vi "Get RX Data Width.vi"(8 "error in":errorcluster, 11 "eye scan in":refnum<class "niHighSpeedSerial Eye Scan v1 Host.lvclass">) -> (0 "error out":errorcluster, 2 "rx internal data width":T1=enum."32 Bit", 3 "eye scan out":refnum<class "niHighSpeedSerial Eye Scan v1 Host.lvclass">)   [LabVIEW 2015, in "niHighSpeedSerial Eye Scan v1 Host.lvclass"]
uses:
  <instrlib>/niHighSpeedSerial/Eye Scan/v1/Host/Eye Scan/niHighSpeedSerial Eye Scan v1 Host.lvclass
  <instrlib>/niHighSpeedSerial/Eye Scan/v1/Host/Common/Public/Data Width.ctl
  <instrlib>/niHighSpeedSerial/Eye Scan/v1/Host/Eye Scan/niHighSpeedSerial Eye Scan v1 Host.lvclass/niHighSpeedSerial Eye Scan v1 Host.ctl
  <vilib>/Utility/error.llb/Error Cluster From Error Code.vi
  <vilib>/ErrorRing/Error Ring.xnode
  <instrlib>/niHighSpeedSerial/Eye Scan/v1/Host/Common/niHighSpeedSerial Eye Scan Common v1 Host.lvlib
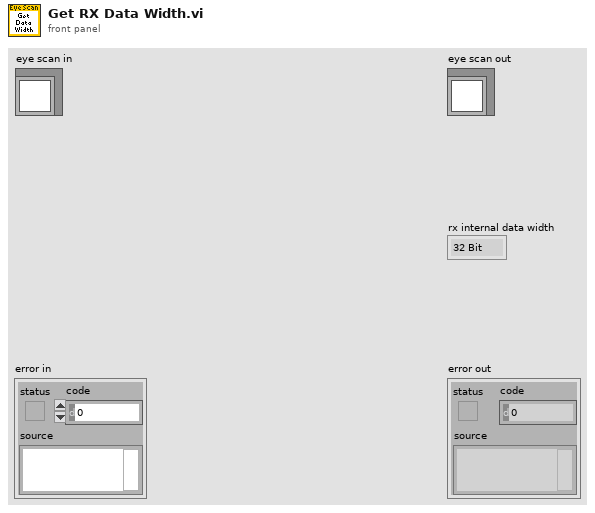
[diagram p1: front panel]
types:
  T1 = typedef "niHighSpeedSerial Eye Scan Common v1 Host.lvlib/Data Width.ctl" = enum16{"16 Bit", "20 Bit", "32 Bit", "40 Bit"}
  T2 = typedef "niHighSpeedSerial Eye Scan v1 Host.lvclass/Private Data.ctl" = cluster{"instruction target":refnum<class "niInstr Instruction Target v1 Host.lvclass">, "channels":T3[], "measure state":T4, "rx output divider":T5, "equalization mode":T6, "rx internal data width":T1, "BER floor":dbl, "number of points completed":i32, "rx output divider configured?":bool, "equalization mode configured?":bool, "rx data width configured?":bool}
  T3 = typedef "niHighSpeedSerial Eye Scan v1 Host.lvclass/Channel Data.ctl" = cluster{"instance":u8, "channel":refnum<class "niHighSpeedSerial Eye Scan Single Point v1 Host.lvclass">, "point iterator":refnum<class "niHighSpeedSerial Eye Scan Point Iterator v1 Host.lvclass">}
  T4 = typedef "niHighSpeedSerial Eye Scan v1 Host.lvclass/Measure State.ctl" = enum16{"Uninitialized", "Initialized", "Ready", "Measuring", "Finished", "Aborted"}
  T5 = typedef "niHighSpeedSerial Eye Scan Common v1 Host.lvlib/RX Output Divider.ctl" = enum16{"1", "2", "4", "8", "16"}
  T6 = typedef "niHighSpeedSerial Eye Scan Common v1 Host.lvlib/Equalization Mode.ctl" = enum16{"DFE", "LPM"}
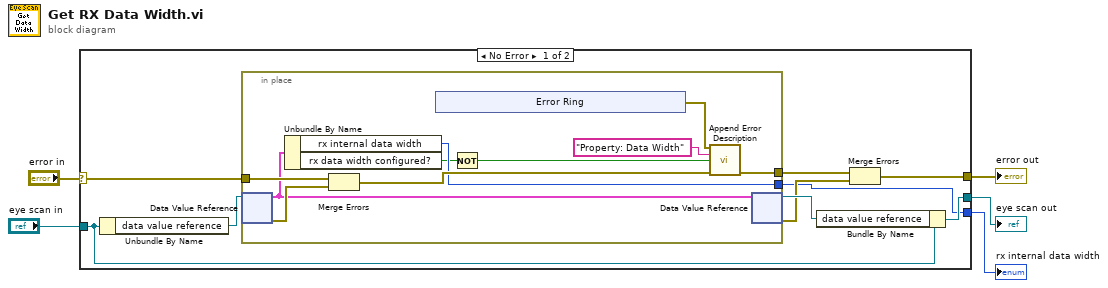
[diagram p0: block diagram]
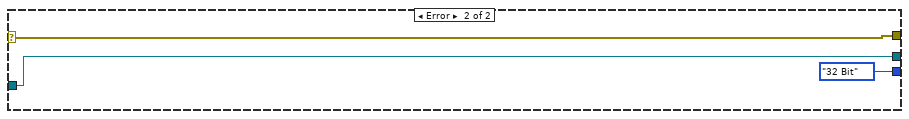
[diagram p2: hidden frame]
diagram:
  n1 = case shown="No Error" "error in" {
    selector: "error in" -> [w10 w31]
    tunnel: [w7 w31] -> w4
    tunnel: [w13 w30] -> w2
    tunnel: "eye scan in" -> [w14 w30]
    tunnel: [w6 Data_Width."32 Bit" ("data width")] -> w1
    frame No Error {
      n2 = Unbundle By Name(w14) -> ("data value reference"=w12:refnum<data-value>)
      n3 = in-place {
        in-place-border: w10 -> [w24]
        in-place-border: [w21] -> w8
        in-place-border: [w19] -> w6
        n4 = in-place-dvr #1(w12) -> (w20:T2, w23:errorcluster)
        n5 = Unbundle By Name(w20) -> ("rx internal data width"=w19:T1, "rx data width configured?"=w16:bool)
        n6 = Merge Errors(w24, w23) -> (w22:errorcluster)
        n7 = xnode "Error Ring"() -> ("error out"=w18:errorcluster)
        n8 = Not(x=w16) -> (.not. x?=w15:bool)
        n9 = call <instrlib>:"Append Error Description.vi"("error to append"=w18, "append string (\"\")"="Property: Data Width" ("replace string (\"\")"), "generate error?"=w15, "error in"=w22) -> ("error out"=w21:errorcluster)  [unwired: 11 in]
        n10 = in-place-dvr #1(w20) -> (w11:refnum<data-value>, w9:errorcluster)
      }
      n11 = Bundle By Name(cluster=w14, "data value reference"=w11) -> (w13:refnum<class "niHighSpeedSerial Eye Scan v1 Host.lvclass">)
      n12 = Merge Errors(w8, w9) -> (w7:errorcluster)
    }
    frame Error {
    }
  }
  "error out" <- w4
  "eye scan out" <- w2
  "rx internal data width" <- w1
